vi "postprocess_stimulus.vi"(4 "Normalize":bool, 6 "Negate":bool, 8 "Bandwidth":dbl=inf format="%0.3f", 9 "Append reversed":bool, 10 "Detrend":bool, 11 "Input":sgl[][](array[numeric])) -> (3 "Output":sgl[][](array[numeric]))   [LabVIEW 2013]
uses:
  <vilib>/Analysis/3filter.llb/Filter Passband Type.ctl
  <vilib>/Analysis/3filter.llb/Zero Phase Filter (Cascade, DBL).vi
  <vilib>/Analysis/NI_AALBase.lvlib
panel:
  # "Remove offset and linear trend."
  # "Make stimulus symmetric by appending a time-reversed  copy. \n If Negate is true, negate the copy also."
  # "Zero phase low-pass filter"
  # "Scale and offset so range is +/- 1."
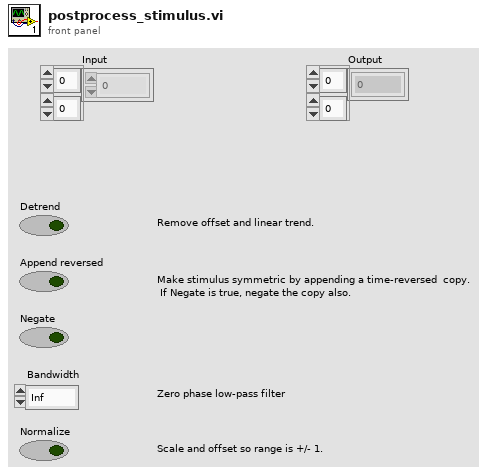
[diagram p1: front panel]
types:
  T1 = typedef "NI_AALBase.lvlib/Filter Passband Type.ctl" = enum32{"Lowpass", "Highpass", "Bandpass", "Bandstop"}
  T2 = cluster{"filter structure":enum32{"IIR 2nd Order", "IIR 4th Order"}, "Reverse Coefficients":dbl[], "Forward Coefficients":dbl[]}
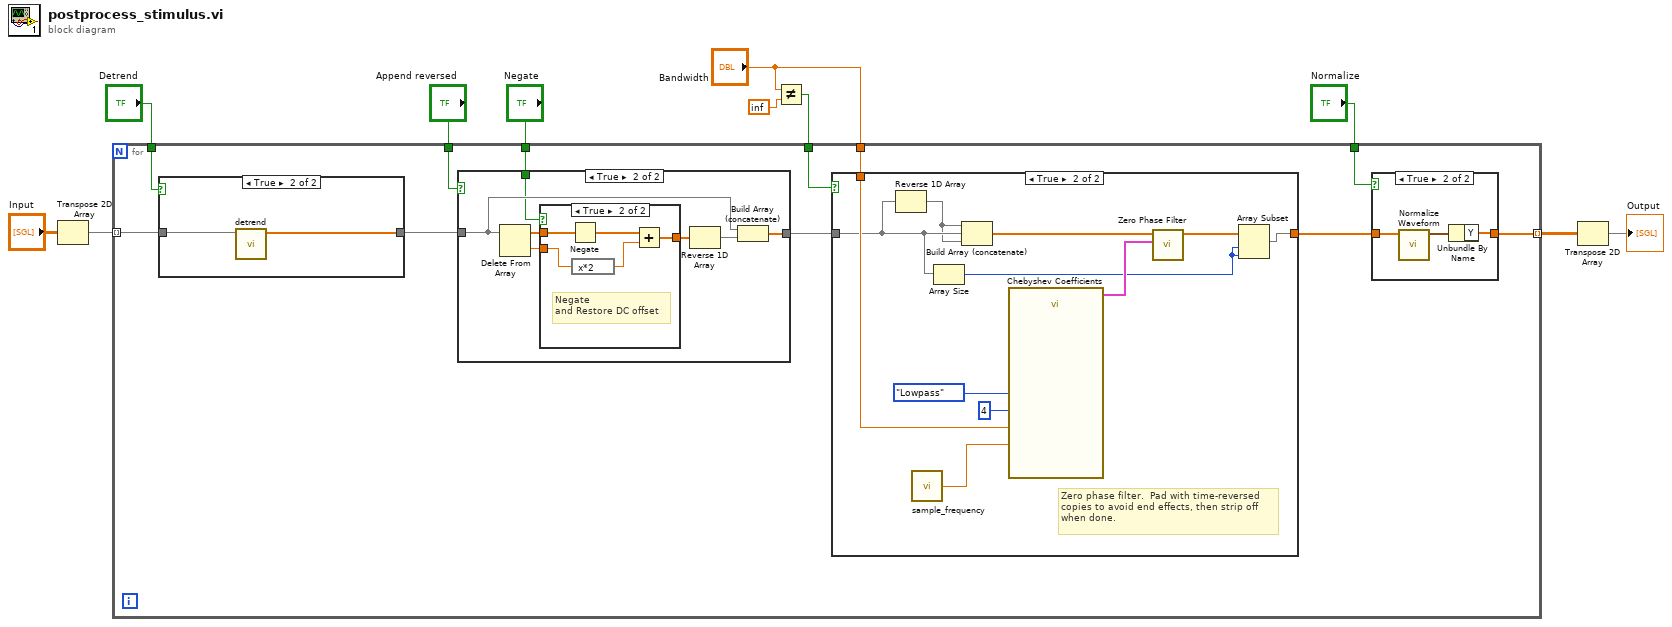
[diagram p0: block diagram]
diagram:
  n1 = Transpose 2D Array(2D array="Input") -> (transposed array=w9:sgl[][])
  n2 = Not Equal?(x="Bandwidth", y=inf) -> (x != y?=w4:bool)
  n3 = for {
    tunnel: w9 -> [w14] mode=indexing
    tunnel: [w16] -> w10 mode=indexing
    tunnel: "Negate" -> [w22]
    tunnel: "Append reversed" -> [w21]
    tunnel: w4 -> [w19]
    tunnel: "Bandwidth" -> [w18]
    tunnel: "Normalize" -> [w15]
    tunnel: "Detrend" -> [w12]
    n4 = case shown="True" w12 {
      tunnel: [w23 w24] -> w13
      tunnel: w14 -> [w23 w25]
      frame False {
      }
      frame True {
        n5 = call "detrend.vi"("Array in"=w25) -> ("Array out"=w24:sgl[])  [unwired: 10 in]
      }
    }
    n6 = case shown="True" w21 {
      tunnel: [w42 w48] -> w20
      tunnel: w13 -> [w42 w44]
      tunnel: w22 -> [_ w43]
      frame False {
      }
      frame True {
        n7 = Delete From Array(array=w44) -> (deleted portion=w46:sgl, array with subset deleted=w47:sgl[])  [unwired: 2 in]
        n8 = case shown="True" w43 {
          tunnel: w47 -> [w50 w55]
          tunnel: w46 -> [_ w54]
          tunnel: [w50 w51] -> w45
          frame False {
          }
          frame True {
            # "Negate\nand Restore DC offset"
            n9 = Negate(x=w55) -> (-x=w53:sgl[])
            n10 = expression code="x*2"(w54) -> (w52:sgl)
            n11 = Add(x=w53, y=w52) -> (x+y=w51:sgl[])
          }
        }
        n12 = Reverse 1D Array(array=w45) -> (reversed array=w49:sgl[])
        n13 = Build Array (concatenate)(w44, w49) -> (w48:sgl[])
      }
    }
    n14 = case shown="True" w19 {
      tunnel: w20 -> [w30 w34]
      tunnel: [w30 w31] -> w17
      tunnel: w18 -> [_ w36]
      frame False {
      }
      frame True {
        # "Zero phase filter.  Pad with time-reversed\ncopies to avoid end effects, then strip off\nwhen done."
        n15 = Reverse 1D Array(array=w34) -> (reversed array=w33:sgl[])
        n16 = call "sample_frequency.vi"() -> ("Sample frequency"=w37:dbl)
        n17 = Array Size(array=w34) -> (size(s)=w35:i32)
        n18 = Build Array (concatenate)(w33, w34, w33) -> (w32:sgl[])
        n19 = call <vilib>:"Chebyshev Coefficients.vi"("order"=4, "filter type"=Filter_Passband_Type."Lowpass", "low cutoff freq: fl"=w36, "sampling freq: fs"=w37) -> ("IIR Filter Cluster"=w40:T2)  [unwired: 6 in, 1 out]
        n20 = call-poly <vilib>:"Zero Phase Filter.vi"("IIR Filter Cluster"=w40, "X"=w32) -> ("Filtered X"=w41:dbl[])  [unwired: 8 in, 1 out]
        n21 = Array Subset(array=w41, index=w35, length=w35) -> (w31:dbl[])
      }
    }
    n22 = case shown="True" w15 {
      tunnel: [w26 w27] -> w16
      tunnel: w17 -> [w26 w28]
      frame False {
      }
      frame True {
        n23 = call <vilib>:"Normalize Waveform.vi"("waveform in"=w28) -> ("normalized waveform"=w29:waveform(dbl))  [unwired: 7 in, 3 out]
        n24 = Unbundle By Name(w29) -> ("Y"=w27:dbl[])
      }
    }
  }
  n25 = Transpose 2D Array(2D array=w10) -> (transposed array=→"Output":dbl[][])
